vi "FilterEmptyLayerIcons.vi"(8 "error in (no error)":errorcluster, 11 "Layers":refnum<class "Layer.lvclass">[](array[class])) -> (0 "error out":errorcluster, 3 "Layers out":refnum<class "Layer.lvclass">[](array[class]), 4 "Remaining Indices":i32[](array[numeric]))   [LabVIEW 2021, in "lv_icon.lvlib"]
doc: "Remove empty (blank) User Layer."
uses:
  <vilib>/LabVIEW Icon API/lv_icon/lv_icon.lvlib
  <vilib>/LabVIEW Icon API/lv_icon/Classes/Layer/Layer.lvclass
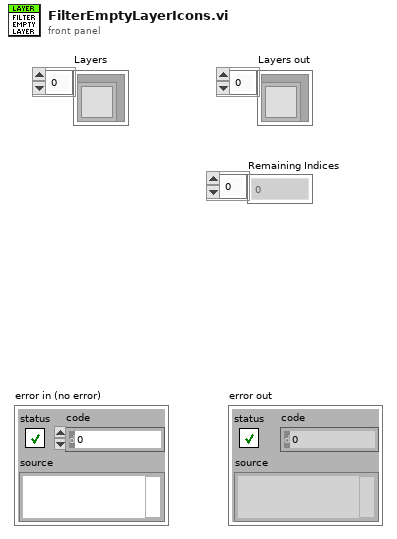
[diagram p1: front panel]
types:
  T1 = cluster{"left":i16, "top":i16, "right":i16, "bottom":i16}
  T2 = typedef "Layer.ctl" = cluster{"LayerIcon":picture, "LayerName":string, "Opacity":u8, "Visibility?":bool}
  T3 = typedef "imagedata.ctl" = cluster{"image type":i32, "image depth":i32, "image":u8[], "mask":u8[], "colors":u32[], "Rectangle":cluster{"left":i16, "top":i16, "right":i16, "bottom":i16}}
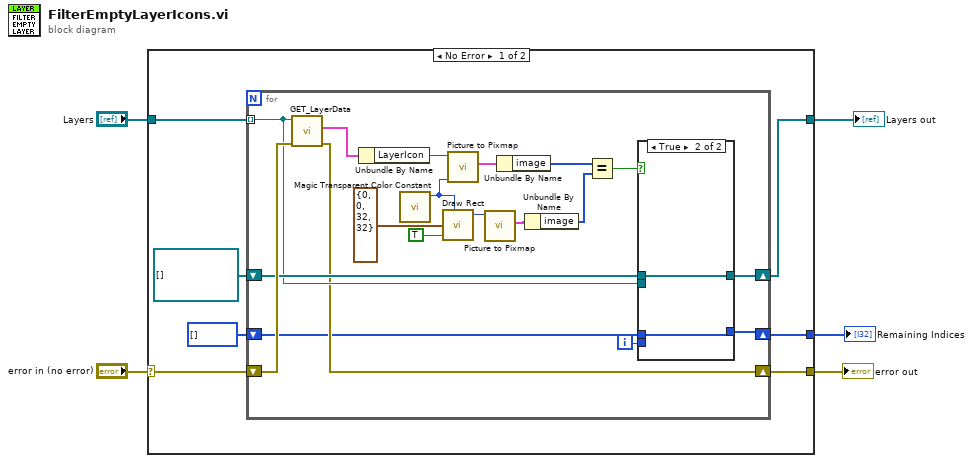
[diagram p0: block diagram]
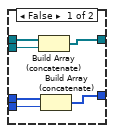
[diagram p2: hidden frame]
diagram:
  n1 = case shown="No Error" "error in (no error)" {
    selector: "error in (no error)" -> [w12 w41]
    tunnel: [w9 w41] -> w4
    tunnel: [w10 w40] -> w2
    tunnel: "Layers" -> [w11 w40]
    tunnel: [w6 _] -> w1
    frame No Error {
      n2 = for {
        tunnel: w11 -> [w27] mode=indexing
        shift-right: [w28] -> w10
        shift-left: refnum<class "Layer.lvclass">[] [] -> [w29]
        shift-right: [w26] -> w9
        shift-left: w12 -> [w31]
        shift-right: [w23] -> w6
        shift-left: i32[] [] -> [w24]
        i -> [w25]
        n3 = call-dynamic "GET_LayerData.vi"("error in (no error)"=w31, "Layer.lvclass in"=w27) -> ("error out"=w26:errorcluster, "Data"=w30:T2)  [unwired: 8 out]
        n4 = Unbundle By Name(w30) -> ("LayerIcon"=w20:picture)
        n5 = call <vilib>:"Magic Transparent Color Constant.vi"() -> ("Magic transparent color constant"=w13:u32)  [unwired: 11 out]
        n6 = call <vilib>:"Draw Rect.vi"("rect"=T1 {"left"=0, "top"=0, "right"=32, "bottom"=32}, "fill?(F)"=TRUE, "color(black)"=w13) -> ("new picture"=w19:picture)  [unwired: 2 in, 4 out]
        n7 = call <vilib>:"Picture to Pixmap.vi"("Background Color"=w13, "picture"=w20) -> ("image data"=w18:T3)  [unwired: 2 in, 7 out]
        n8 = call <vilib>:"Picture to Pixmap.vi"("picture"=w19) -> ("image data"=w17:T3)  [unwired: 3 in, 7 out]
        n9 = Unbundle By Name(w18) -> ("image"=w15:u8[])
        n10 = Unbundle By Name(w17) -> ("image"=w14:u8[])
        n11 = Equal?(x=w15, y=w14) -> (x = y?=w16:bool)
        n12 = case shown="True" w16 {
          tunnel: w29 -> [w37 w39]
          tunnel: [w35 w39] -> w28
          tunnel: w27 -> [w36 _]
          tunnel: w25 -> [w34 _]
          tunnel: w24 -> [w33 w38]
          tunnel: [w32 w38] -> w23
          frame False {
            n13 = Build Array (concatenate)(w37, w36) -> (w35:refnum<class "Layer.lvclass">[])
            n14 = Build Array (concatenate)(w33, w34) -> (w32:i32[])
          }
          frame True {
          }
        }
      }
    }
    frame Error {
    }
  }
  "error out" <- w4
  "Layers out" <- w2
  "Remaining Indices" <- w1
